vi "Error.vi"(8 "error in":errorcluster, 11 "Ignore Errors (Runtime)":i32[](array[numeric])) -> (0 "error out":errorcluster)   [LabVIEW 2014]
uses:
  Message Queue/Message Queue.lvlib
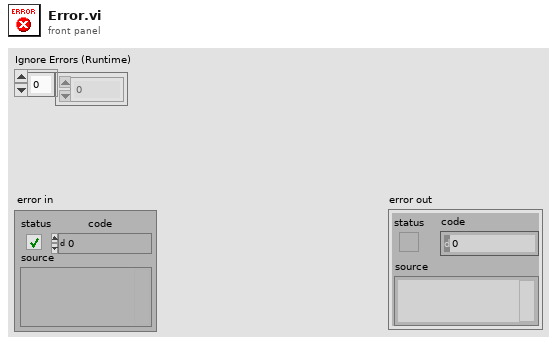
[diagram p1: front panel]
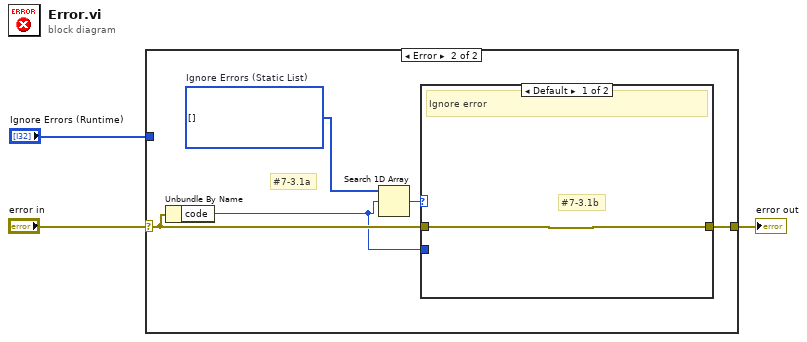
[diagram p0: block diagram]
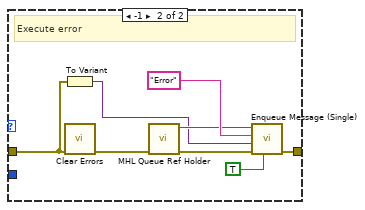
[diagram p3: hidden frame]
diagram:
  n1 = case shown="Error" "error in" {
    selector: "error in" -> [w4 w8]
    tunnel: [w4 w9] -> w3
    tunnel: "Ignore Errors (Runtime)" -> [_ _]
    frame No Error {
    }
    frame Error {
      w5 = i32[] []  # Ignore Errors (Static List)
      # "#7-3.1a"
      n2 = Unbundle By Name(w8) -> ("code"=w6:i32)
      n3 = Search 1D Array(1D array=w5, element=w6) -> (index of element=w7:i32)  [unwired: 1 in]
      n4 = case shown="Default" w7 {
        tunnel: w8 -> [w10 w13]
        tunnel: [w10 w11] -> w9
        tunnel: w6 -> [_ _]
        frame Default {
          # "#7-3.1b"
          # "Ignore error"
        }
        frame -1 {
          # "Execute error"
          n5 = To Variant(anything=w13) -> (Variant=w15:variant)
          n6 = call <vilib>:"Clear Errors.vi"("error in (no error)"=w13) -> ("error out"=w12:errorcluster)  [unwired: 5 in, 1 out]
          n7 = call "MHL Queue Ref Holder.vi"("error in"=w12) -> ("error out"=w16:errorcluster, "Input Message Queue"=w17:refnum<queue>)  [unwired: 9 in]
          n8 = call "Enqueue Message (Single).vi"("Priority Message? (F)"=TRUE, "error in (no error)"=w16, "Message Data"=w15, "Message"="Error", "Message Queue"=w17) -> ("error out"=w11:errorcluster)  [unwired: 5 in, 1 out]
        }
      }
    }
  }
  "error out" <- w3
